vi "Play Previous Song.vi"(8 "error in (no error)":errorcluster, 11 "SongQueueActor In":refnum<class "SongQueueActor.lvclass">) -> (0 "error out":errorcluster, 3 "SongQueueActor Out":refnum<class "SongQueueActor.lvclass">)   [LabVIEW 2015, in "SongQueueActor.lvlib" / "SongQueueActor.lvclass"]
uses:
  SongQueueActor.lvclass
  SongQueueActor.lvclass/SongQueueActor.ctl
  file/MusicElement/MusicElementLibrary/MusicElementLibrary.lvclass/MusicElementLibrary.ctl
  controls/Queue Song Display.ctl
  file/MusicElement/Song/Song Duration.ctl
  controls/Dequeue Control.ctl
  builds/xctls/Song Queue/Song Queue.lvlibp/app/xctls/SongQueue/Song Queue.xctl
  file/MusicElement/MusicElement.lvclass
  SongPlayerActor/SongPlayerActor Messages/Play Song Msg/Play Song Msg.lvclass
  file/MusicElement/Song/Song.lvclass
  file/MusicElement/MusicElementLibrary/MusicElementLibrary.lvclass
  AlbumImageActor/AlbumImageActor Messages/Download Album Image Msg/Download Album Image Msg.lvclass
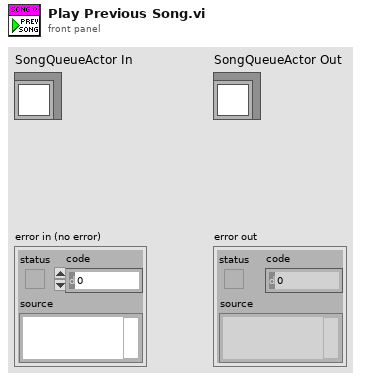
[diagram p1: front panel]
types:
  T1 = typedef "Queue Song Display.ctl" = cluster{"Song Name":string, "Artist":string, "Album":string, "Duration (s)":T2, "UID":string, "Dequeue":T3}
  T2 = typedef "Song.lvclass/Song Duration.ctl" = timestamp
  T3 = typedef "Dequeue Control.ctl" = bool
  T4 = typedef "Song Queue.lvlibp/Queue Song Display.ctl" = cluster{"Song Name":string, "Artist":string, "Album":string, "Duration (s)":T5, "UID":string, "Dequeue":T6}
  T5 = typedef "Song Queue.lvlibp/Song.lvclass/Song Duration.ctl" = timestamp
  T6 = typedef "Song Queue.lvlibp/Dequeue Control.ctl" = bool
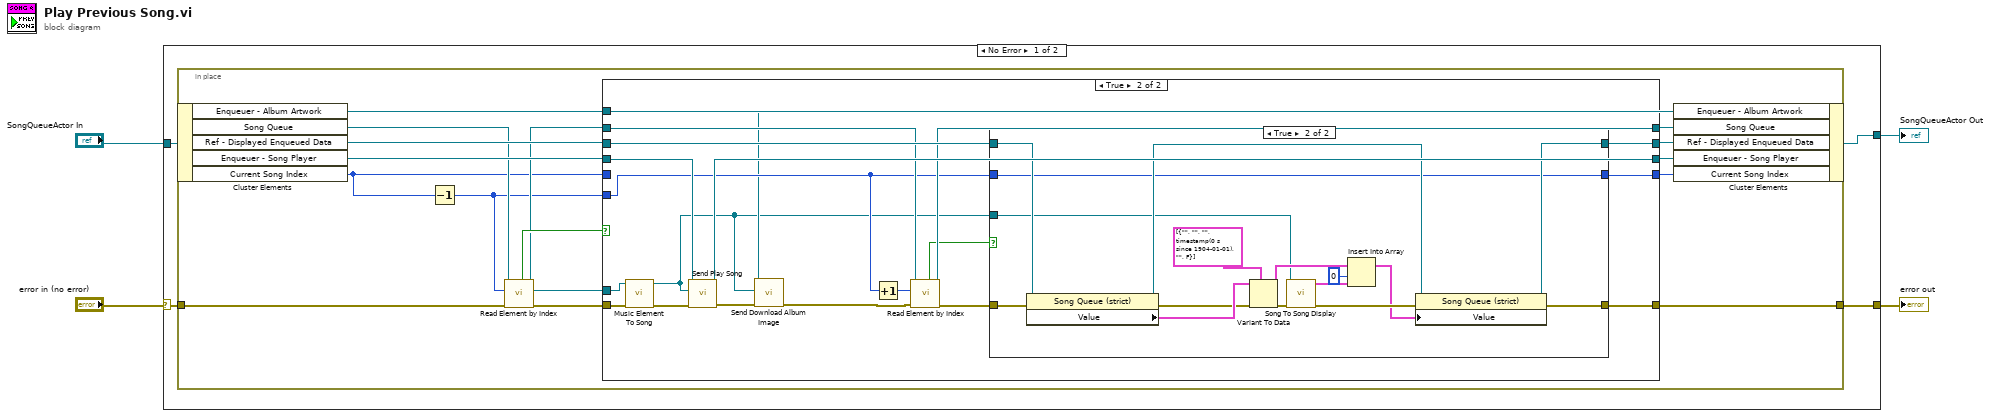
[diagram p0: block diagram]
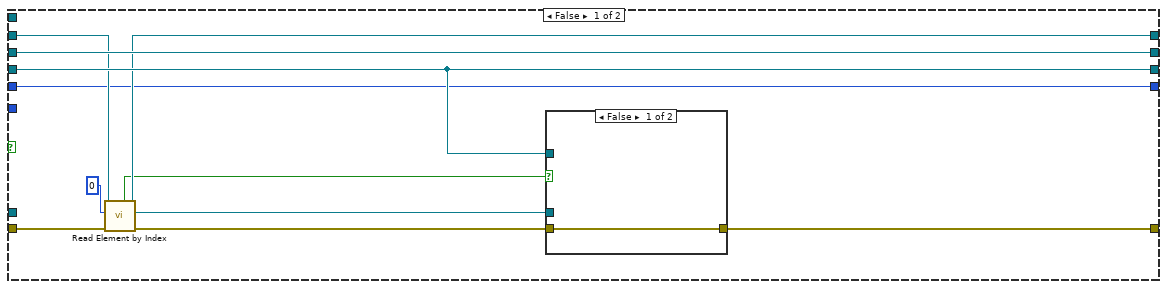
[diagram p2: hidden frame]
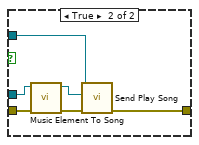
[diagram p3: hidden frame]
diagram:
  n1 = case shown="No Error" "error in (no error)" {
    selector: "error in (no error)" -> [w7 w82]
    tunnel: [w5 w82] -> w3
    tunnel: [w6 w81] -> w2
    tunnel: "SongQueueActor In" -> [w8 w81]
    frame No Error {
      n2 = in-place {
        in-place-border: w7 -> [w17]
        in-place-border: [w22] -> w5
        n3 = in-place-cluster #1(w8) -> ("Enqueuer - Album Artwork"=w9:refnum<class "Message Enqueuer.lvclass">, "Song Queue"=w12:refnum<class "SongLibrary.lvclass">, "Ref - Displayed Enqueued Data"=w20:refnum<vi>, "Enqueuer - Song Player"=w24:refnum<class "Message Enqueuer.lvclass">, "Current Song Index"=w11:i32)
        n4 = Decrement(x=w11) -> (x-1=w10:i32)
        n5 = call "Read Element by Index.vi"("error in (no error)"=w17, "index"=w10, "MusicElementLibrary in"=w12) -> ("error out"=w14:errorcluster, "MusicElement.lvclass"=w13:refnum<class "MusicElement.lvclass">, "MusicElementLibrary out"=w15:refnum<class "SongLibrary.lvclass">, "Found?"=w16:bool)  [unwired: 5 in]
        n6 = case shown="True" w16 {
          tunnel: w14 -> [w32 w50]
          tunnel: w24 -> [w33 w61]
          tunnel: [w33 w60] -> w23
          tunnel: [w34 w59] -> w22
          tunnel: w11 -> [w25 _]
          tunnel: [w25 w56] -> w21
          tunnel: w20 -> [w35 w58]
          tunnel: [w35 w57] -> w19
          tunnel: [w30 w52] -> w18
          tunnel: w15 -> [w31 w53]
          tunnel: w13 -> [_ w49]
          tunnel: w10 -> [_ w47]
          tunnel: w9 -> [_ w44]
          frame False {
            n7 = call "Read Element by Index.vi"("error in (no error)"=w32, "index"=0 ("Index"), "MusicElementLibrary in"=w31) -> ("error out"=w26:errorcluster, "MusicElement.lvclass"=w27:refnum<class "MusicElement.lvclass">, "MusicElementLibrary out"=w30:refnum<class "SongLibrary.lvclass">, "Found?"=w29:bool)  [unwired: 5 in]
            n8 = case shown="False" w29 {
              tunnel: w26 -> [w36 w38]
              tunnel: [w36 w42] -> w34
              tunnel: w33 -> [_ w41]
              tunnel: w27 -> [_ w37]
              frame False {
              }
              frame True {
                n9 = call "Music Element To Song.vi"("error in (no error)"=w38, "MusicElement"=w37) -> ("error out"=w40:errorcluster, "Song out"=w39:refnum<class "Song.lvclass">)  [unwired: 8 in]
                n10 = call "Send Play Song.vi"("error in (no error)"=w40, "Song"=w39, "Message Enqueuer in"=w41) -> ("error out"=w42:errorcluster)  [unwired: 7 in, 1 out]
              }
            }
          }
          frame True {
            n11 = call "Music Element To Song.vi"("error in (no error)"=w50, "MusicElement"=w49) -> ("error out"=w48:errorcluster, "Song out"=w43:refnum<class "Song.lvclass">)  [unwired: 8 in]
            n12 = call "Send Play Song.vi"("error in (no error)"=w48, "Song"=w43, "Message Enqueuer in"=w61) -> ("error out"=w46:errorcluster, "Message Enqueuer out"=w60:refnum<class "Message Enqueuer.lvclass">)  [unwired: 7 in]
            n13 = call "Send Download Album Image.vi"("error in (no error)"=w46, "Song"=w43, "Message Enqueuer in"=w44) -> ("error out"=w45:errorcluster)  [unwired: 7 in, 1 out]
            n14 = Increment(x=w47) -> (x+1=w55:i32)
            n15 = call "Read Element by Index.vi"("error in (no error)"=w45, "index"=w55, "MusicElementLibrary in"=w53) -> ("error out"=w54:errorcluster, "MusicElementLibrary out"=w52:refnum<class "SongLibrary.lvclass">, "Found?"=w51:bool)  [unwired: 5 in, 1 out]
            n16 = case shown="True" w51 {
              tunnel: w54 -> [w63 w71]
              tunnel: [w63 w70] -> w59
              tunnel: w58 -> [w64 w69]
              tunnel: [w64 w67] -> w57
              tunnel: w43 -> [_ w66]
              tunnel: [w62 w65] -> w56
              tunnel: w47 -> [w62 w65]
              frame False {
              }
              frame True {
                n17 = property class="Song Queue (strict)"(reference=w69, error in=w71) -> (reference out=w68:refnum<vi>, error out=w72:errorcluster, "Value"=w73:T4[])
                n18 = Variant To Data(error in=w72, type=T1[] [{"Song Name"="", "Artist"="", "Album"="", "Duration (s)"=timestamp(0 s since 1904-01-01), "UID"="", "Dequeue"=FALSE}], Variant=w73) -> (data=w80:T1[], error out=w79:errorcluster)
                n19 = call "Song To Song Display.vi"("error in (no error)"=w79, "Song"=w66) -> ("error out"=w77:errorcluster, "Song DIsplay"=w75:T1)  [unwired: 8 in]
                n20 = Insert Into Array(array=w80, index=0, new element=w75) -> (w76:T1[])
                n21 = property class="Song Queue (strict)"(reference=w68, error in=w77, "Value"=w76) -> (reference out=w67:refnum<vi>, error out=w70:errorcluster)
              }
            }
          }
        }
        n22 = in-place-cluster #1("Enqueuer - Album Artwork"=w9, "Song Queue"=w18, "Ref - Displayed Enqueued Data"=w19, "Enqueuer - Song Player"=w23, "Current Song Index"=w21) -> (w6:refnum<class "SongQueueActor.lvclass">)
      }
    }
    frame Error {
    }
  }
  "error out" <- w3
  "SongQueueActor Out" <- w2
